vi "Get PID gains.vi"(0 "PID parameters":cluster{"Kp":dbl, "Ti":dbl, "Td":dbl} {"Td" format="%.2f"; "Ti" format="%.2f"; "Kp" format="%.2f"}, 1 "options":T1={"sp low"=0.0, "sp high"=100.0, "out low"=-100.0, "out high"=100.0, "hold (F)"=FALSE, "auto (T)"=TRUE, "pro. band (F)"=FALSE, "reverse acting (T)"=TRUE, "beta"=1.0, "linearity"=1.0, "dt (s)"=-1.0} {"dt (s)" format="%.2f"; "linearity" min=0.0 max=1.0 format="%.2f"; "sp low" format="%.2f"; "sp high" format="%.2f"; "out low" format="%.2f"; "out high" format="%.2f"; "beta" min=0.0 max=1.0 format="%.2f"}) -> (2 "Kc":dbl format="%.4f", 3 "Ki":dbl format="%.4f", 4 "Kd":dbl format="%.4f")   [LabVIEW 2020, in "NI_PID__prctrl compat.lvlib"]
doc: "This VI determines the gains to be used for the proportional, derivative and integral action of the controller."
uses:
  <vilib>/addons/control/pid/NI_PID__prctrl compat.lvlib
panel:
  # "Proportional gain or band (Kc)"
  # "Integral (reset) time (Ti, min)"
  # "Derivative (rate) time (Td, min)"
  # "SP & PV range:"
  # "Output range:"
  # "-1: default,using\nsystem clock"
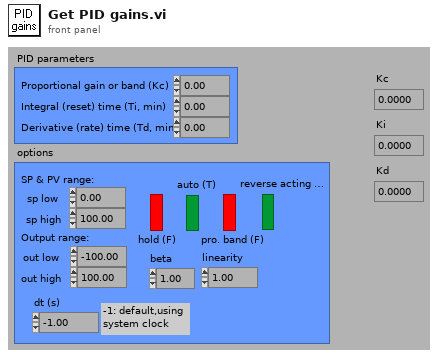
[diagram p1: front panel]
types:
  T1 = cluster{"sp low":dbl, "sp high":dbl, "out low":dbl, "out high":dbl, "hold (F)":bool, "auto (T)":bool, "pro. band (F)":bool, "reverse acting (T)":bool, "beta":dbl, "linearity":dbl, "dt (s)":dbl}
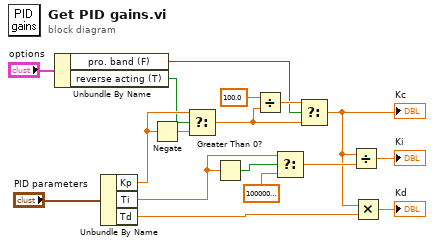
[diagram p0: block diagram]
diagram:
  n1 = Unbundle By Name("options") -> ("pro. band (F)"=w8:bool, "reverse acting (T)"=w9:bool)
  n2 = Unbundle By Name("PID parameters") -> ("Kp"=w14:dbl, "Ti"=w11:dbl, "Td"=w3:dbl)
  n3 = Negate(x=w14) -> (-x=w17:dbl)
  n4 = Select(t=w14, s=w9, f=w17) -> (s? t:f=w10:dbl)
  n5 = Greater Than 0?(x=w11) -> (x > 0?=w13:bool)
  n6 = Divide(x=100.0, y=w10) -> (x/y=w15:dbl)
  n7 = Select(t=w11, s=w13, f=10000000000.0) -> (s? t:f=w7:dbl)
  n8 = Select(t=w15, s=w8, f=w10) -> (s? t:f=w1:dbl)
  "Kc" <- w1
  n9 = Divide(x=w1, y=w7) -> (x/y=→"Ki":dbl)
  n10 = Multiply(x=w1, y=w3) -> (x*y=→"Kd":dbl)
